vi "GFITS_SeparateHeaders.vi"(0 "number of before keys":i32[](array[numeric]), 1 "Database RefNum in":T1, 2 "ref":u64, 5 "mext":bool, 7 "number of Extensions":u16, 9 "Keywords":string[][][](array[string]), 11 "error in (no error)":errorcluster, 13 "headers":bool=TRUE) -> (10 "expID":string, 15 "error out":errorcluster)   [LabVIEW 2016]
uses:
  DBSHAND/private/vis/DatabaseHand_RefNum.ctl
  GFITS_Gbls.vi
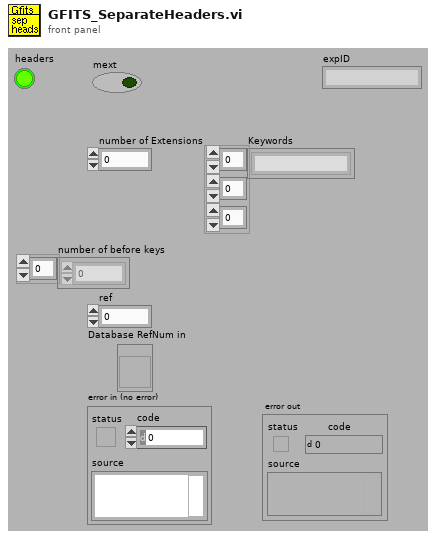
[diagram p1: front panel]
types:
  T1 = typedef "DatabaseHand_RefNum.ctl" = refnum<vi>
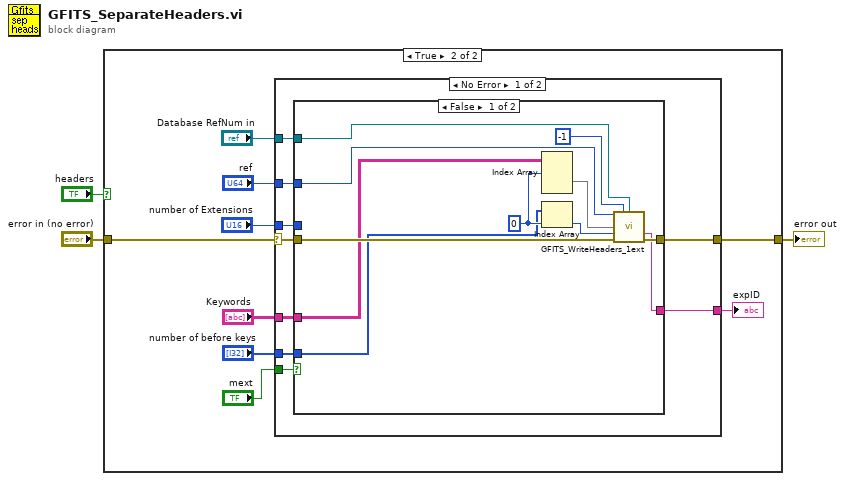
[diagram p0: block diagram]
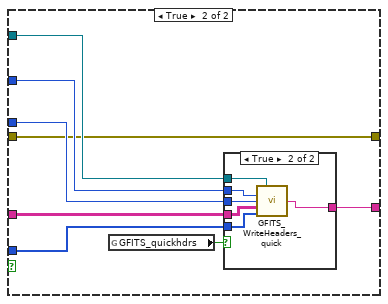
[diagram p3: hidden frame]
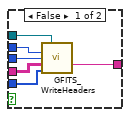
[diagram p4: hidden frame]
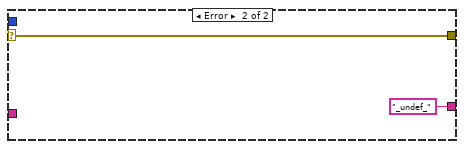
[diagram p5: hidden frame]
diagram:
  n1 = case shown="True" "headers" {
    tunnel: "error in (no error)" -> [w4 w9]
    tunnel: [w4 w7] -> w2
    frame False {
    }
    frame True {
      n2 = case shown="No Error" w9 {
        selector: w9 -> [w17 w55]
        tunnel: "mext" -> [w22 _]
        tunnel: "number of Extensions" -> [w21 _]
        tunnel: "ref" -> [w20 _]
        tunnel: [w19 w55] -> w7
        tunnel: "Database RefNum in" -> [w18 _]
        tunnel: [w16 "_undef_" ("expID")] -> w8
        tunnel: "Keywords" -> [w15 _]
        tunnel: "number of before keys" -> [w14 _]
        frame No Error {
          n3 = case shown="False" w22 {
            tunnel: w21 -> [_ w39]
            tunnel: w20 -> [w33 w40]
            tunnel: w18 -> [w32 w41]
            tunnel: w17 -> [w31 w38]
            tunnel: [w30 w38] -> w19
            tunnel: [w29 w37] -> w16
            tunnel: w15 -> [w27 w36]
            tunnel: w14 -> [w24 w35]
            frame False {
              w25 = 0 ("index (page)")
              n4 = Index Array(array=w27, index (dim 0)=w25) -> (element=w26:string[][])  [unwired: 2 in]
              n5 = Index Array(array=w24, index=w25) -> (element=w23:i32)
              n6 = call "GFITS_WriteHeaders_1ext.vi"("ref"=w33, "extension"=-1, "Database RefNum in"=w32, "Keywords"=w26, "numer of keywords"=w23, "error in (no error)"=w31) -> ("expID"=w29:string, "error out"=w30:errorcluster)  [unwired: 1 in, 7 out]
            }
            frame True {
              n7 = global read "GFITS_Gbls.vi" "GFITS_quickhdrs"() -> (w34:bool)
              n8 = case shown="True" w34 {
                tunnel: w41 -> [w47 w53]
                tunnel: w40 -> [w46 w52]
                tunnel: w39 -> [w45 w51]
                tunnel: w35 -> [w44 w50]
                tunnel: [w43 w49] -> w37
                tunnel: w36 -> [w42 w48]
                frame False {
                  n9 = call "GFITS_WriteHeaders.vi"("Database RefNum in"=w47, "ref"=w46, "number of extensions"=w45, "Keywords"=w42, "number of keywords"=w44) -> ("expID"=w43:string)  [unwired: 1 in, 9 out]
                }
                frame True {
                  n10 = call "GFITS_WriteHeaders_quick.vi"("Database RefNum in"=w53, "ref"=w52, "number of extensions"=w51, "Keywords"=w48, "number of keywords"=w50) -> ("expID"=w49:string)  [unwired: 1 in, 9 out]
                }
              }
            }
          }
        }
        frame Error {
        }
      }
      "expID" <- w8
    }
  }
  "error out" <- w2
